vi "close.vi"(8 "error in (no error)":errorcluster caption="错误输入（无错误）", 11 "EPEVER-MPPT 输入":refnum<class "EPEVER-MPPT.lvclass">) -> (0 "error out":errorcluster caption="错误输出", 3 "EPEVER-MPPT 输出":refnum<class "EPEVER-MPPT.lvclass">)   [LabVIEW 2016, in "EPEVER-MPPT.lvlib" / "EPEVER-MPPT.lvclass"]
uses:
  EPEVER-MPPT.lvclass
  EPEVER-MPPT.lvclass/EPEVER-MPPT.ctl
  <vilib>/Plasmionique/MB Master/MB_Master/MB_Master.lvclass
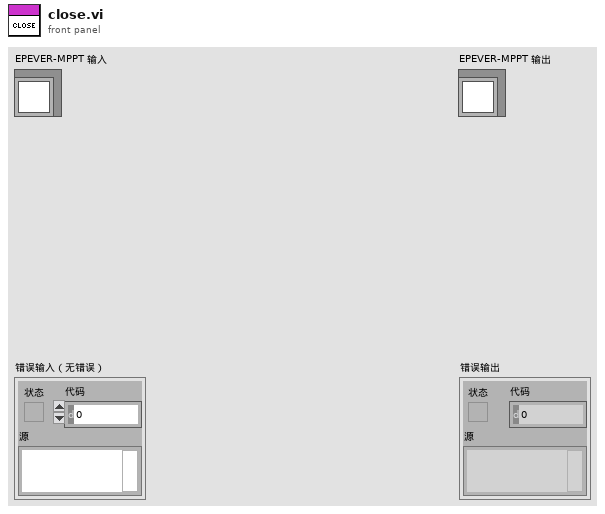
[diagram p1: front panel]
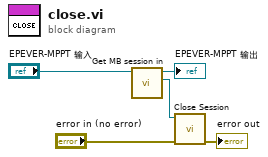
[diagram p0: block diagram]
diagram:
  n1 = call "Get MB session in.vi"("EPEVER-MPPT in"="EPEVER-MPPT 输入") -> ("MB Serial Master:MB_Master"=w3:refnum<class "MB_Master.lvclass">, "EPEVER-MPPT out"=→"EPEVER-MPPT 输出":refnum<class "EPEVER-MPPT.lvclass">)  [unwired: 9 in]
  n2 = call-dynamic "Close Session.vi"("error in (no error)"="error in (no error)", "MB session in"=w3) -> ("error out"=→"error out":errorcluster)  [unwired: 9 in]
